vi "Log AO AI.vi"(8 "error in (no error)":errorcluster, 11 "Instrument.Lockin in":refnum<class "Instrument.Lockin.lvclass">) -> (0 "error out":errorcluster)   [LabVIEW 2019, in "Instrument.Lockin.lvlib" / "Instrument.Lockin.lvclass"]
uses:
  Instrument.Lockin.lvclass
  C:/Program Files (x86)/National Instruments/LabVIEW 2019/user.lib/LevyLab/Instrument Framework/Instrument/Instrument.lvclass
  Instrument.Lockin.lvclass/Instrument.Lockin.ctl
  <userlib>/LevyLab/Instrument Framework/Instrument/Instrument.lvclass
  Instrument.DAQ/Instrument.DAQ.lvclass
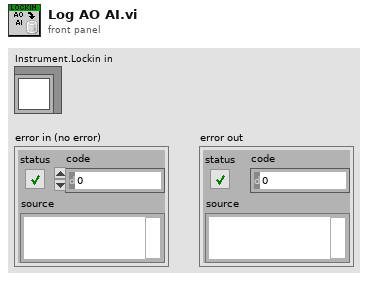
[diagram p1: front panel]
types:
  T1 = typedef "Instrument.Lockin.lvlib/Instrument.DAQ.lvclass/DeviceInfo--Cluster.ctl" = cluster{"DeviceName":string, "DevIsSimulated":bool, "DeviceSerialNumber":u32, "ProductType":string, "ProductCategory":i32, "ProductNumber":u32, "ChassisNumber":u32, "SlotNumber":u32, "ChassisName":string, "ChassisSerialNumber":u32}
  T2 = cluster{"ChassisSerialNumber":u32, "AI Channel":i32, dbl, bool}
  T3 = cluster{"ChassisSerialNumber":u32, "AO Channel":i32, dbl, bool}
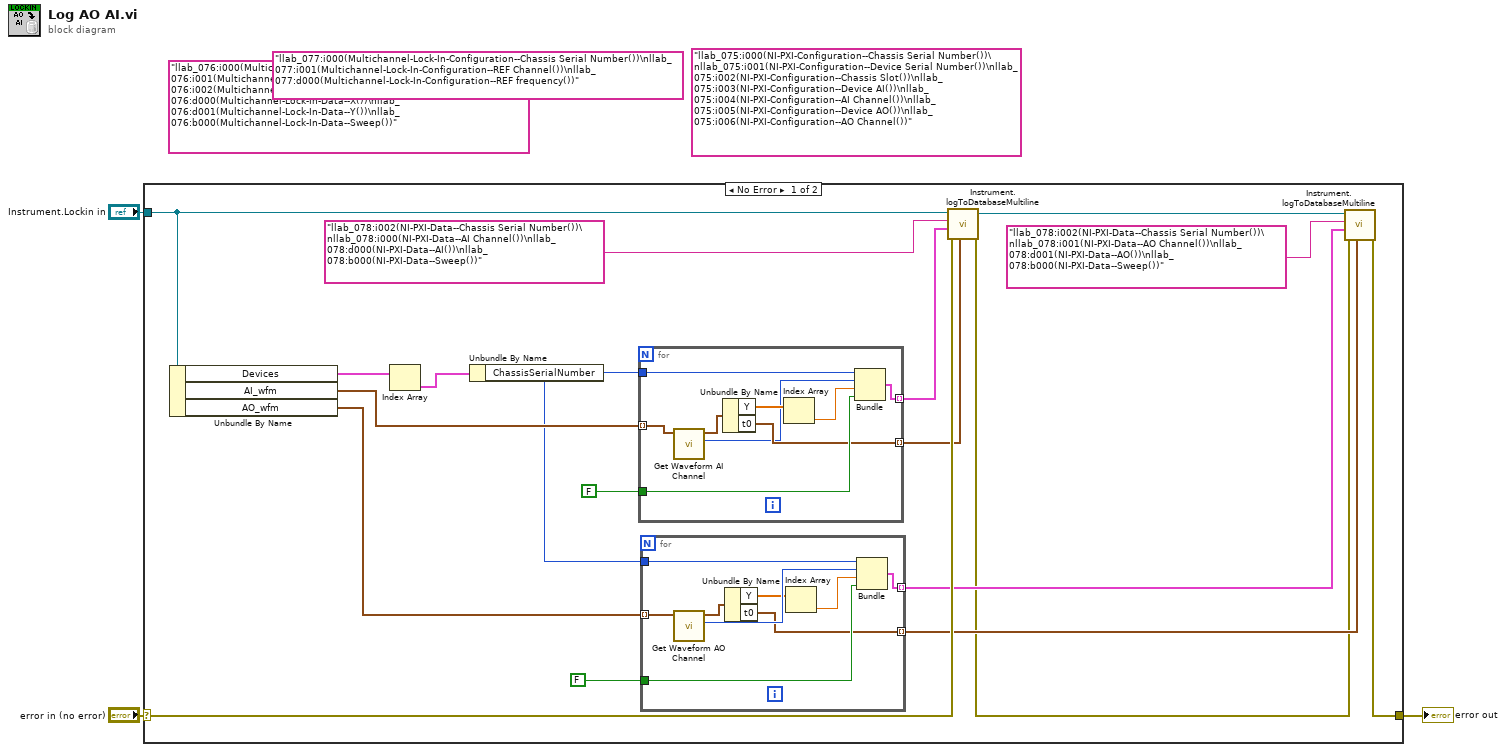
[diagram p0: block diagram]
diagram:
  (unwired) "llab_076:i000(Multichannel-Lock-In-Data--Chassis Serial Number())\nllab_076:i001(Multichannel-Lock-In-Data--AI Channel())\nllab_076:i002(Multichannel-Lock-In-Data--REF Channel())\nllab_076:d000(Multichannel-Lock-In-Data--X())\nllab_076:d001(Multichannel-Lock-In-Data--Y())\nllab_076:b000(Multichannel-Lock-In-Data--Sweep())"
  (unwired) "llab_075:i000(NI-PXI-Configuration--Chassis Serial Number())\nllab_075:i001(NI-PXI-Configuration--Device Serial Number())\nllab_075:i002(NI-PXI-Configuration--Chassis Slot())\nllab_075:i003(NI-PXI-Configuration--Device AI())\nllab_075:i004(NI-PXI-Configuration--AI Channel())\nllab_075:i005(NI-PXI-Configuration--Device AO())\nllab_075:i006(NI-PXI-Configuration--AO Channel())"
  (unwired) "llab_077:i000(Multichannel-Lock-In-Configuration--Chassis Serial Number())\nllab_077:i001(Multichannel-Lock-In-Configuration--REF Channel())\nllab_077:d000(Multichannel-Lock-In-Configuration--REF frequency())"
  n1 = case shown="No Error" "error in (no error)" {
    selector: "error in (no error)" -> [w19 w40]
    tunnel: "Instrument.Lockin in" -> [w21 _]
    tunnel: [w20 w40] -> w2
    frame No Error {
      n2 = Unbundle By Name(w21) -> ("Devices"=w18:T1[], "AI_wfm"=w13:waveform(dbl)[], "AO_wfm"=w4:waveform(dbl)[])
      n3 = Index Array(array=w18) -> (element=w14:T1)  [unwired: 1 in]
      n4 = Unbundle By Name(w14) -> ("ChassisSerialNumber"=w7:u32)
      n5 = for {
        tunnel: w7 -> [w39]
        tunnel: [w38] -> w17 mode=indexing
        tunnel: [w34] -> w16 mode=indexing
        tunnel: w13 -> [w33] mode=indexing
        tunnel: FALSE -> [w35]
        n6 = call "Get Waveform AI Channel.vi"("Reference in"=w33) -> ("AI Channel"=w31:i32, "Reference out"=w32:waveform(dbl))  [unwired: 8 in, 1 out]
        n7 = Unbundle By Name(w32) -> ("Y"=w37:dbl[], "t0"=w34:timestamp)
        n8 = Index Array(array=w37) -> (element=w36:dbl)  [unwired: 1 in]
        n9 = Bundle("ChassisSerialNumber"=w39, "AI Channel"=w31, w36, w35) -> (w38:T2)  [unwired: 1 in]
      }
      n10 = for {
        tunnel: w7 -> [w30]
        tunnel: [w29] -> w10 mode=indexing
        tunnel: [w22] -> w11 mode=indexing
        tunnel: w4 -> [w28] mode=indexing
        tunnel: FALSE -> [w24]
        n11 = call "Get Waveform AO Channel.vi"("Reference in"=w28) -> ("AO Channel"=w27:i32, "Reference out"=w23:waveform(dbl))  [unwired: 8 in, 1 out]
        n12 = Unbundle By Name(w23) -> ("Y"=w26:dbl[], "t0"=w22:timestamp)
        n13 = Index Array(array=w26) -> (element=w25:dbl)  [unwired: 1 in]
        n14 = Bundle("ChassisSerialNumber"=w30, "AO Channel"=w27, w25, w24) -> (w29:T3)  [unwired: 1 in]
      }
      n15 = call <userlib>:"Instrument.logToDatabaseMultiline.vi"("timestamps"=w16, "error in (no error)"=w19, "Data"=w17, "Paths"="llab_078:i002(NI-PXI-Data--Chassis Serial Number())\nllab_078:i000(NI-PXI-Data--AI Channel())\nllab_078:d000(NI-PXI-Data--AI())\nllab_078:b000(NI-PXI-Data--Sweep())", "Instrument"=w21) -> ("error out"=w5:errorcluster, "Instrument out"=w9:refnum<class "Instrument.Lockin.lvclass">)  [unwired: 5 in]
      n16 = call <userlib>:"Instrument.logToDatabaseMultiline.vi"("timestamps"=w11, "error in (no error)"=w5, "Data"=w10, "Paths"="llab_078:i002(NI-PXI-Data--Chassis Serial Number())\nllab_078:i001(NI-PXI-Data--AO Channel())\nllab_078:d001(NI-PXI-Data--AO())\nllab_078:b000(NI-PXI-Data--Sweep())", "Instrument"=w9) -> ("error out"=w20:errorcluster)  [unwired: 5 in, 1 out]
    }
    frame Error {
    }
  }
  "error out" <- w2
